vi "参数设置页.vi"() -> ()   [LabVIEW 2016, in "斯坦道氨氮.lvlib"]
uses:
  <vilib>/Plasmionique/MB Master/MB_Master/MB_Master.lvclass
  <vilib>/ptbypt/NI_PtbyPt.lvlib
panel:
  out "数据刷新时间":string
  in  "通讯连接":bool
  out "MB table":enum32{"Serial", "TCP"}(tab)
  in  "请选择串口:":refnum<visa-resource-name>
  in  "IP":string="127.0.0.1"
  in  "PORT":string="1001"
  in  "通信方式选择":enum16{"串口", "TCP"}(ring)
  in  "盐度自动补偿：":bool
  out "盐度补偿值":dbl caption="盐度补偿值："
  in  "刷新":bool
  in  "测量模式":enum16{"水样测量", "零点核查", "跨度核查", "标样核查", "加标回收"}(ring)
  in  "参数下拉列表":u16(ring)
  in  "量程下拉列表":enum16{"低量程", "高量程"}(ring)
  in  "流程路径":path=path "data/流程.xml"
  in  "标样核查量程模式":enum16{"高量程", "低量程", "自动"}(ring) caption="标样核查量程模式："
  in  "加标回收量程模式":enum16{"高量程", "低量程", "自动"}(ring) caption="加标回收量程模式："
  in  "跨度核查量程模式":enum16{"高量程", "低量程", "自动"}(ring) caption="跨度核查量程模式："
  in  "零点核查量程模式":enum16{"高量程", "低量程", "自动"}(ring) caption="零点核查量程模式："
  in  "水样测试量程模式":enum16{"高量程", "低量程", "自动"}(ring) caption="水样测试量程模式："
  out "稀释度":dbl caption="稀释度："
  out "阈值（高->低）":dbl caption="阈值（高->低）："
  out "阈值（低->高）":dbl caption="阈值（低->高）："
  out "量程下限":dbl caption="量程下限："
  out "量程上限":dbl caption="量程上限："
  out "检出限":dbl caption="检出限："
  out "曲线截距":dbl caption="曲线截距：" format="%#.6f"
  out "曲线斜率":dbl caption="曲线斜率：" format="%#.6f"
  out "二次多项式系数":dbl caption="二次多项式系数：" format="%#.6f"
  out "消解时长":dbl caption="消解时长："
  out "消解温度":dbl caption="消解温度："
  out "测量精度":u16 caption="测量精度："
  in  "标样核查标液浓度":dbl caption="标样核查标液浓度："
  in  "跨度核查标液浓度":dbl caption="跨度核查标液浓度："
  in  "零点核查标液浓度":dbl caption="零点核查标液浓度："
  in  "跨度值":dbl caption="跨度值："
  # "ppt"
  # "mg/L"
  # "mg/L"
  # "mg/L"
  # "mg/L"
  # "mg/L"
  # "min"
  # "℃"
  # "mg/L"
  # "mg/L"
  # "mg/L"
  # "mg/L"
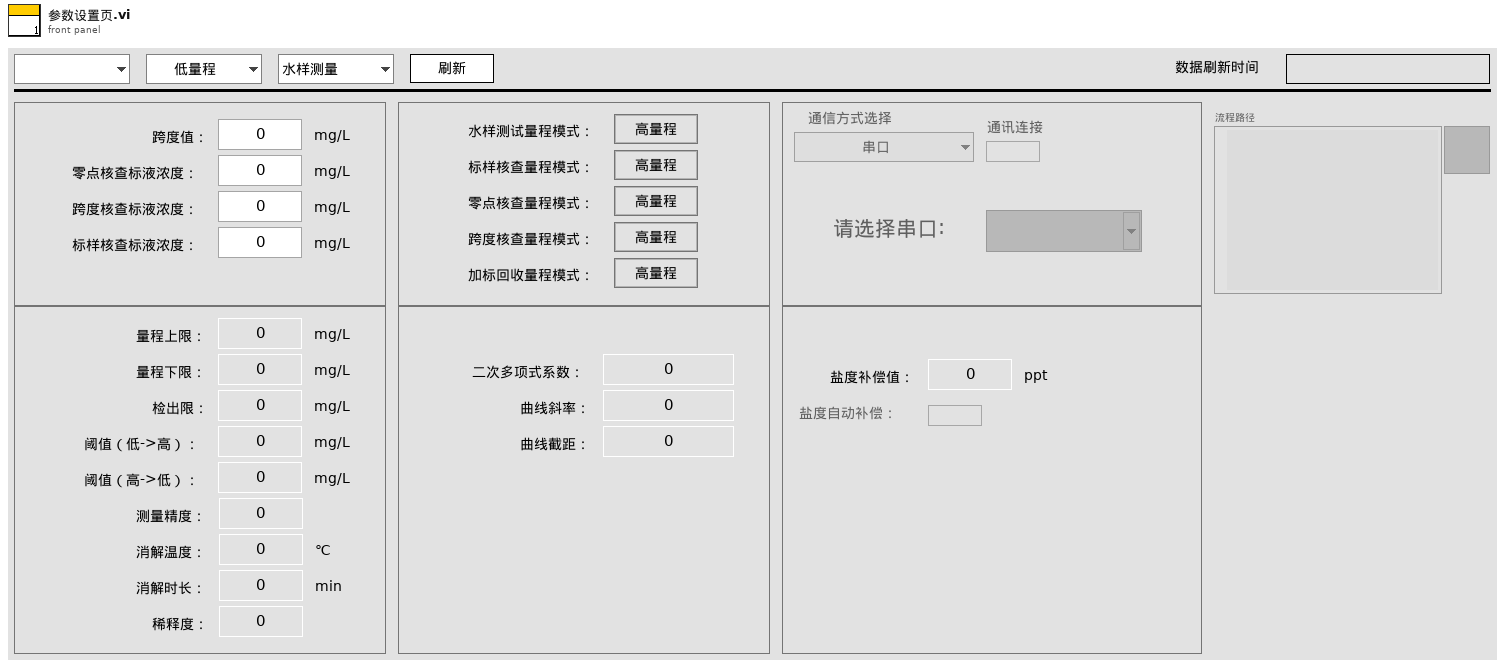
[diagram p1: front panel]
types:
  T1 = typedef "LVStringsAndValuesArrayTypeDef_U16.ctl" = cluster{"String":string, "Value":u16}[]
  T2 = enum8{"Enabled", "Disabled", "Disabled and Grayed Out"}
  T3 = cluster{"标液浓度1":dbl, "测量吸光度1":dbl, "样品1启用":bool, "标液浓度2":dbl, "测量吸光度2":dbl, "样品2启用":bool, "标液浓度3":dbl, "测量吸光度3":dbl, "样品3启用":bool, "标液浓度4":dbl, "测量吸光度4":dbl, "样品4启用":bool, "标液浓度5":dbl, "测量吸光度5":dbl, "样品5启用":bool, "模型":enum32{"线性", "多项式"}, "精度":dbl, "XY图":cluster{"X Values":dbl[], "Y Values":dbl[]}[], "拟合公式":string, "r^2":dbl, "标样一校准时间":timestamp, "标样二校准时间":timestamp, "标样三校准时间":timestamp, "标样四校准时间":timestamp, "标样五校准时间":timestamp, "二次方程":cluster{"c":dbl, "x":dbl, "x^2":dbl}, "标定时间":timestamp}
  T4 = cluster{"系统时间":timestamp, "工作状态":u16, "测量模式":enum16{"待机", "连续模式", "周期模式", "定点模式", "受控模式", "手动模式"}, "告警代码":u16, "故障代码":u16, "日志代码":u16, "软件版本":u16, "F0":sgl, "F1":sgl, "F2":sgl, "F3":sgl, "T":sgl, "H":sgl, "id":u16, "flowid":u16, "量程":u16, "总磷控温温度1":sgl, "营养盐控温温度2":sgl, "ADC":sgl}
  T5 = cluster{"测量精度":u16, "检出限":dbl, "上限":dbl, "下限":dbl, "阈值（低->高）":dbl, "阈值（高->低）":dbl, "稀释度":dbl}
  T6 = cluster{"泵类型":u8, "进样速度":u32, "出样速度":u32, "泵阀量":u8, "光谱仪类型":u8, "光谱采样次数":u8, "氙灯次数":u8, "B":u16, "C":u16, "D":u16, "E":u16, "B_COD":u16, "C_COD":u16, "D_COD":u16, "E_COD":u16, "G":u16, "M":u16, "N":u16, "氨氮注射泵控温下限":sgl, "氨氮注射泵控温上限":sgl, "总氮注射泵控温下限":sgl, "总氮注射泵控温上限":sgl, "消解温度下限":sgl, "消解温度上限":sgl, "加热10s限值":sgl, "高温高压阀开阀温度":sgl, "总氮x公式0":u8, "总氮x公式1":sgl, "总氮x公式2":sgl, "总磷浊度稀释系数":sgl, "总磷浊度补偿权重1":sgl, "总磷浊度补偿权重2":sgl, "盐度系数":sgl, "氨氮补偿系数1":sgl, "氨氮补偿系数2":sgl}
  T7 = cluster{"标液浓度1":dbl, "测量吸光度1":dbl, "样品1启用":bool, "标液浓度2":dbl, "测量吸光度2":dbl, "样品2启用":bool, "标液浓度3":dbl, "测量吸光度3":dbl, "样品3启用":bool, "标液浓度4":dbl, "测量吸光度4":dbl, "样品4启用":bool, "标液浓度5":dbl, "测量吸光度5":dbl, "样品5启用":bool, "模型":enum32{"线性", "多项式"}, "精度":dbl, "XY图":cluster{"X Values":dbl[], "Y Values":dbl[]}[], "拟合公式":string, "r^2":dbl, "标样一校准时间":timestamp, "标样二校准时间":timestamp, "标样三校准时间":timestamp, "标样四校准时间":timestamp, "标样五校准时间":timestamp, "二次方程":cluster{"c":dbl, "x":dbl, "x^2":dbl}, "标定时间":timestamp}[][]
  T8 = typedef "斯坦道氨氮.lvlib/关键参数.ctl" = cluster{"测量量程":sgl, "测量检出限":sgl, "测量精度":sgl, "测量间隔":sgl, "消解温度":sgl, "消解时长":sgl, "三项式系数":sgl, "二次多项式系数":sgl, "曲线斜率":sgl, "曲线截距":sgl, "线性相关系数":sgl, "空白校准时间":timestamp, "标样校准时间":timestamp, "测量信号值":sgl, "稀释倍数":sgl, "量程系数":sgl}
  T9 = cluster{"水样测试量程模式":enum16{"高量程", "低量程", "自动"}, "零点核查量程模式":enum16{"高量程", "低量程", "自动"}, "跨度核查量程模式":enum16{"高量程", "低量程", "自动"}, "加标回收量程模式":enum16{"高量程", "低量程", "自动"}, "标样核查量程模式":enum16{"高量程", "低量程", "自动"}}
  T10 = cluster{"总磷跨度值":dbl, "总磷零点标准液浓度":dbl, "总磷跨度标准液浓度":dbl, "总磷标准液标准浓度":dbl, "总氮跨度值":dbl, "总氮零点标准液浓度":dbl, "总氮跨度标准液浓度":dbl, "总氮标准液标准浓度":dbl, "COD跨度值":dbl, "COD零点标准液浓度":dbl, "COD跨度标准液浓度":dbl, "COD标准液标准浓度":dbl, "氨氮跨度值":dbl, "氨氮零点标准液浓度":dbl, "氨氮跨度标准液浓度":dbl, "氨氮标准液标准浓度":dbl, "磷酸盐跨度值":dbl, "磷酸盐零点标准液浓度":dbl, "磷酸盐跨度标准液浓度":dbl, "磷酸盐标准液标准浓度":dbl, "硝氮跨度值":dbl, "硝氮零点标准液浓度":dbl, "硝氮跨度标准液浓度":dbl, "硝氮标准液标准浓度":dbl, "亚硝氮跨度值":dbl, "亚硝氮零点标准液浓度":dbl, "亚硝氮跨度标准液浓度":dbl, "亚硝氮标准液标准浓度":dbl, "硫化物跨度值":dbl, "硫化物零点标准液浓度":dbl, "硫化物跨度标准液浓度":dbl, "硫化物标准液标准浓度":dbl, "硅酸盐跨度值":dbl, "硅酸盐零点标准液浓度":dbl, "硅酸盐跨度标准液浓度":dbl, "硅酸盐标准液标准浓度":dbl}
  T11 = cluster{"水样测试量程模式":u16, "零点核查量程模式":u16, "跨度核查量程模式":u16, "加标回收量程模式":u16, "标样核查量程模式":u16}
  T12 = cluster{"水样测试量程模式":enum16{"H", "L", "AUTO"}, "空白核查量程模式":enum16{"H", "L", "AUTO"}, "跨度核查量程模式":enum16{"H", "L", "AUTO"}, "加标回收量程模式":enum16{"H", "L", "AUTO"}, "标样核查量程模式":enum16{"H", "L", "AUTO"}}
  T13 = cluster{"水样测试量程模式":u16, "空白核查量程模式":u16, "跨度核查量程模式":u16, "加标回收量程模式":u16, "标样核查量程模式":u16}
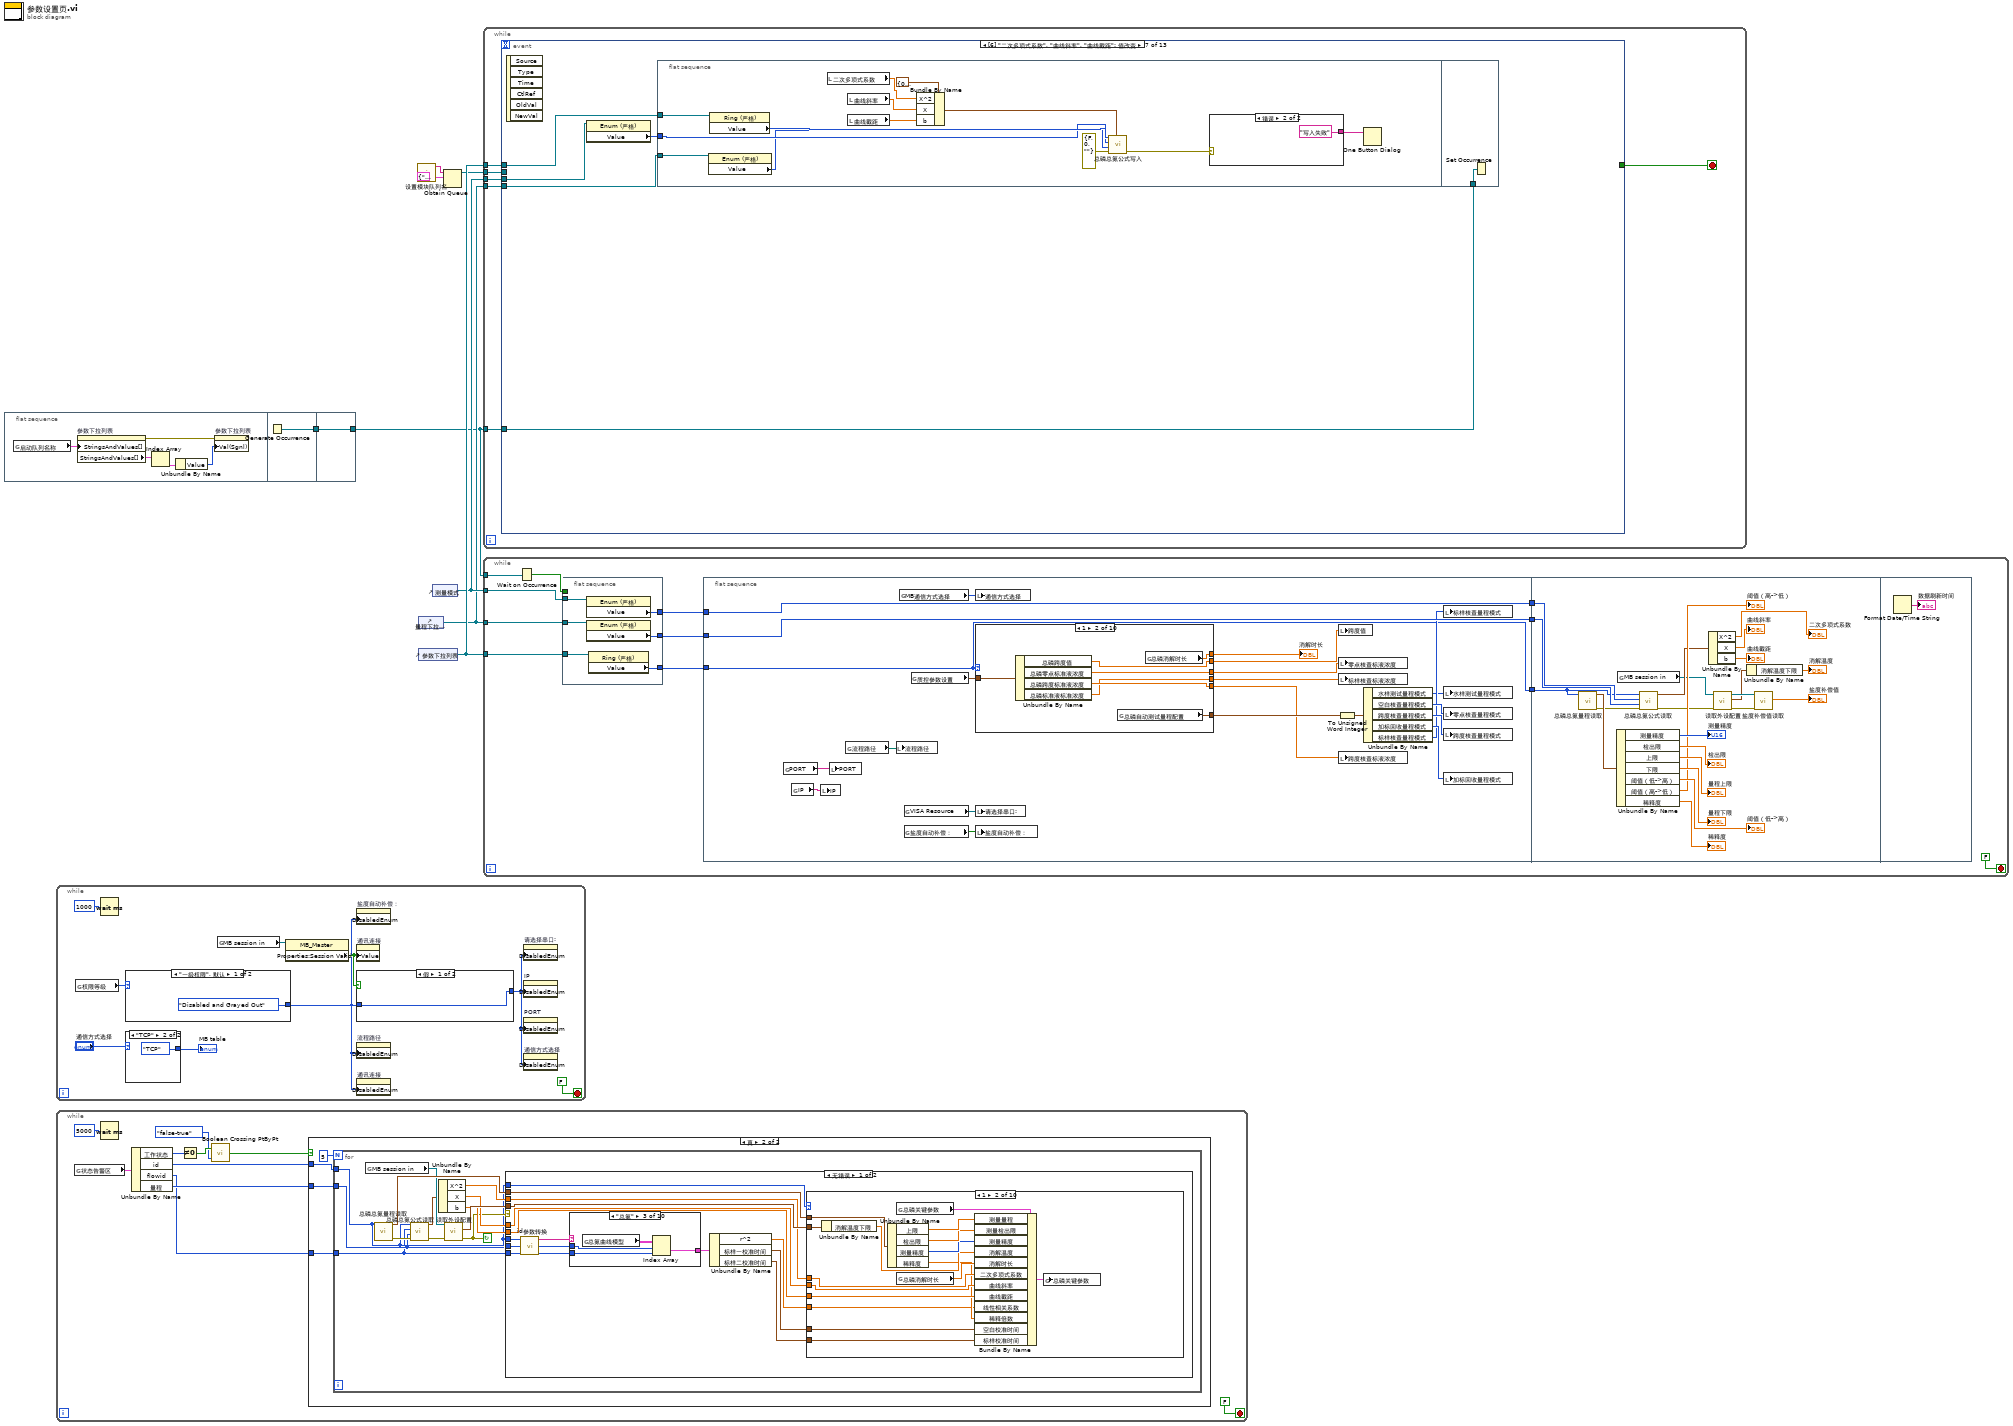
[diagram p0: block diagram]
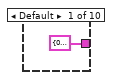
[diagram p3: hidden frame]
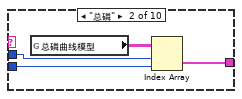
[diagram p4: hidden frame]
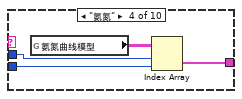
[diagram p5: hidden frame]
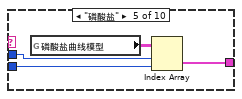
[diagram p6: hidden frame]
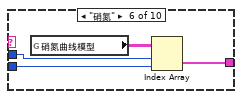
[diagram p7: hidden frame]
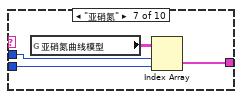
[diagram p8: hidden frame]
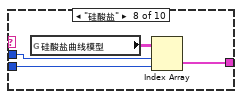
[diagram p9: hidden frame]
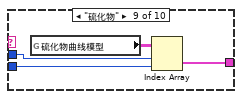
[diagram p10: hidden frame]
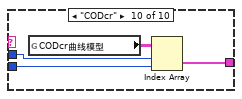
[diagram p11: hidden frame]
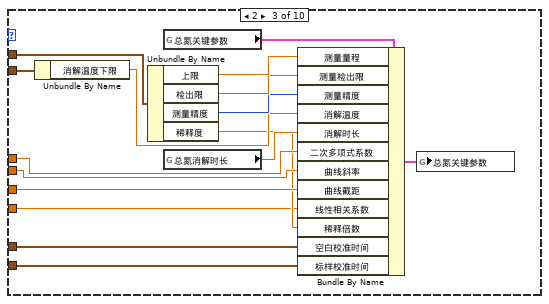
[diagram p13: hidden frame]
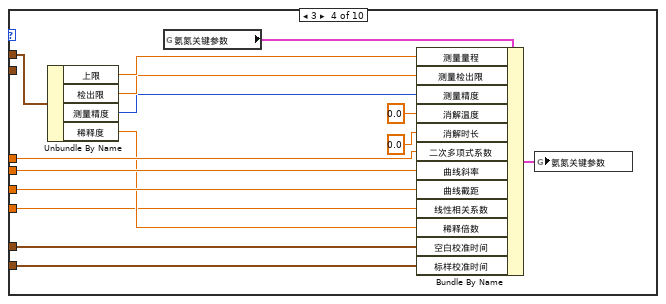
[diagram p14: hidden frame]
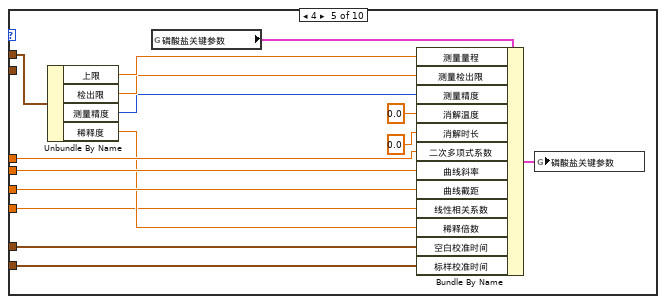
[diagram p15: hidden frame]
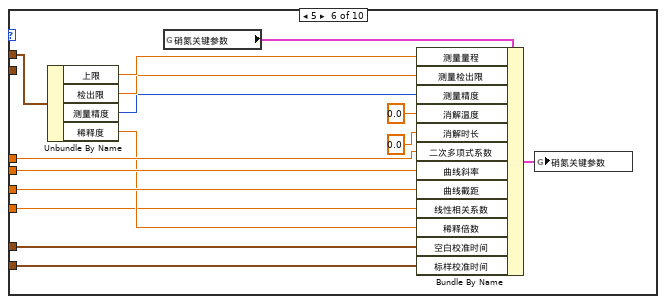
[diagram p16: hidden frame]
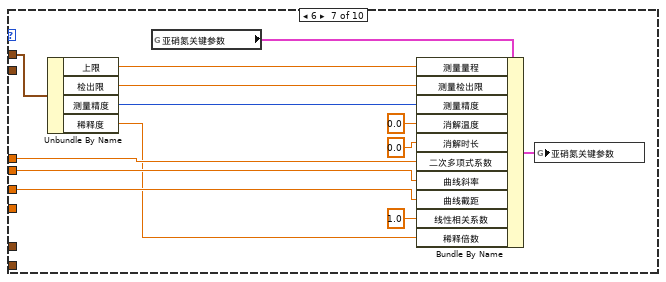
[diagram p17: hidden frame]
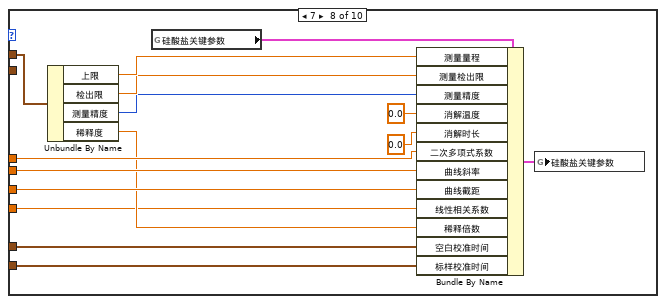
[diagram p18: hidden frame]
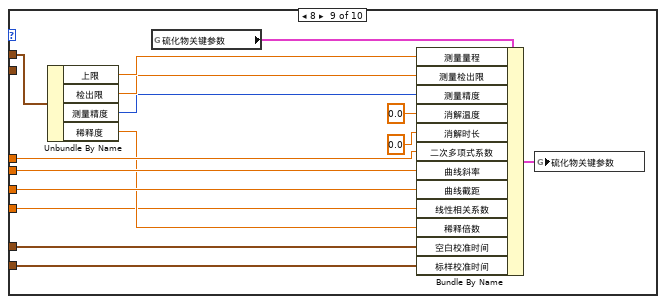
[diagram p19: hidden frame]
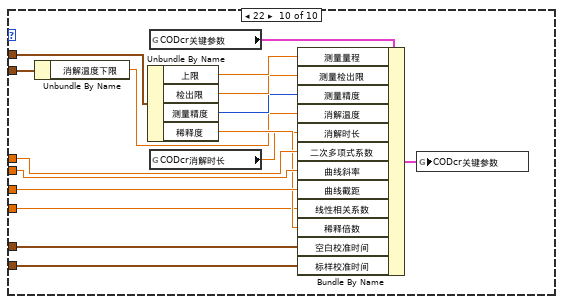
[diagram p20: hidden frame]
diagram:
  n1 = flat-sequence {
    tunnel: [w14] -> w7
    tunnel: [w15] -> w1
    tunnel: w7 -> [w15]
    frame #0 {
      n2 = global read "总磷总氮断电保存全局变量.vi" "启动队列名称"() -> (w9:cluster{"String":string, "Value":u16}[])
      n3 = property on="参数下拉列表" class="Ring (严格)"("StringsAndValues[]"=w9) -> (error out=w12:errorcluster, "StringsAndValues[]"=w10:T1)  [unwired: 2 in, 1 out]
      n4 = Index Array(array=w10) -> (element=w11:cluster{"String":string, "Value":u16})  [unwired: 1 in]
      n5 = Unbundle By Name(w11) -> ("Value"=w13:u16)
      n6 = property on="参数下拉列表" class="Ring (严格)"(error in=w12, "Val(Sgnl)"=w13) -> ()  [unwired: 1 in, 2 out]
    }
    frame #1 {
      n7 = Generate Occurrence() -> (w14:refnum<k4>)
    }
    frame #2 {
    }
  }
  n8 = while {
    stop <- FALSE stop-if-true
    n9 = global read "VAR总磷总氮全局变量.vi" "权限等级"() -> (w16:enum16{"一级权限", "二级权限", "三级权限", "超级权限"})
    n10 = Wait (ms)(milliseconds to wait=u32 1000 ("等待时间（毫秒）")) -> ()  [unwired: 1 out]
    n11 = case shown="\"一级权限\", 默认" w16 {
      tunnel: [T2."Disabled and Grayed Out" ("禁用") T2."Enabled" ("禁用")] -> w17
      frame "一级权限", Default {
      }
      frame "二级权限".."超级权限" {
      }
    }
    n12 = case shown="\"TCP\"" "通信方式选择" {
      tunnel: [enum32{"Serial", "TCP"}."Serial" ("MB table") enum32{"Serial", "TCP"}."TCP" ("MB table")] -> w19
      frame "串口", Default {
      }
      frame "TCP" {
      }
    }
    "MB table" <- w19
    n13 = global read "VAR总磷总氮全局变量.vi" "MB session in"() -> (w23:refnum<class "MB_Master.lvclass">)
    n14 = property class="MB_Master"(reference=w23) -> ("Properties:Session Valid"=w21:bool)  [unwired: 1 in, 2 out]
    n15 = property on="盐度自动补偿：" class="Bool (严格)"("DisabledEnum"=w17) -> ()  [unwired: 2 in, 2 out]
    n16 = property on="通讯连接" class="Bool (严格)"("Value"=w21) -> ()  [unwired: 2 in, 2 out]
    n17 = case shown="假" w21 {
      tunnel: [w29 T2."Disabled and Grayed Out" ("禁用")] -> w20
      tunnel: w17 -> [w29 _]
      frame False {
      }
      frame True {
      }
    }
    n18 = property on="流程路径" class="Path"("DisabledEnum"=w17) -> ()  [unwired: 2 in, 2 out]
    n19 = property on="通讯连接" class="Bool (严格)"("DisabledEnum"=w17) -> ()  [unwired: 2 in, 2 out]
    n20 = property on="请选择串口:" class="VISAName"("DisabledEnum"=w20) -> ()  [unwired: 2 in, 2 out]
    n21 = property on="IP" class="Str"("DisabledEnum"=w20) -> ()  [unwired: 2 in, 2 out]
    n22 = property on="PORT" class="Str"("DisabledEnum"=w20) -> ()  [unwired: 2 in, 2 out]
    n23 = property on="通信方式选择" class="Enum (严格)"("DisabledEnum"=w20) -> ()  [unwired: 2 in, 2 out]
  }
  n24 = while {
    stop <- FALSE stop-if-true
    n25 = global read "VAR总磷总氮全局变量.vi" "状态告警区"() -> (w40:T4)
    n26 = Wait (ms)(milliseconds to wait=u32 5000 ("等待时间（毫秒）")) -> ()  [unwired: 1 out]
    n27 = Unbundle By Name(w40) -> ("工作状态"=w36:u16, "id"=w37:u16, "flowid"=w38:u16, "量程"=w39:u16)
    n28 = Not Equal To 0?(x=w36) -> (x != 0?=w35:bool)
    n29 = call <vilib>:"Boolean Crossing PtByPt.vi"("direction"=enum16{"either", "false-true", "true-false"}."false-true", "input"=w35) -> ("crossing"=w33:bool)  [unwired: 1 in]
    n30 = case shown="真" w33 {
      tunnel: w39 -> [_ w44]
      tunnel: w38 -> [_ w43]
      tunnel: w37 -> [_ w42]
      frame False {
      }
      frame True {
        n31 = for {
          N: 5 -> [_]
          tunnel: w44 -> [w46]
          tunnel: w43 -> [w45]
          tunnel: w42 -> [w47]
          stop <- w48 continue-if-true
          n32 = global read "VAR总磷总氮全局变量.vi" "MB session in"() -> (w56:refnum<class "MB_Master.lvclass">)
          n33 = call "总磷总氮量程读取.vi"("测量参数"=w47) -> ("error out"=w50:errorcluster, "量程参数读取"=w57:T5)  [unwired: 9 in]
          n34 = call "总磷总氮公式读取.vi"("error in (no error)"=w50, "量程"=w46, "测量模式"=w45, "测量参数"=w47) -> ("error out"=w49:errorcluster, "公式"=w54:cluster{"X^2":dbl, "X":dbl, "b":dbl})  [unwired: 6 in]
          n35 = Unbundle By Name(w54) -> ("X^2"=w53:dbl, "X"=w52:dbl, "b"=w51:dbl)
          n36 = call "读取外设配置.vi"("error in (no error)"=w49, "MB session in"=w56) -> ("error out"=w48:errorcluster, "外设配置"=w55:T6)  [unwired: 7 in, 1 out]
          n37 = case shown="无错误" w48 {
            tunnel: w57 -> [w71 _]
            tunnel: w55 -> [w70 _]
            tunnel: w53 -> [w69 _]
            tunnel: w52 -> [w68 _]
            tunnel: w51 -> [w67 _]
            tunnel: w47 -> [w66 _]
            tunnel: w47 -> [w63 _]
            tunnel: w46 -> [w62 _]
            tunnel: w45 -> [w61 _]
            frame No Error {
              n38 = call "id参数转换.vi"("id"=w63) -> ("table输出"=w65:string)  [unwired: 9 in, 1 out]
              n39 = case shown="\"总氮\"" w65 {
                tunnel: w61 -> [_ w75 w77 w82 w86 w90 w94 w98 w102 w106]
                tunnel: w62 -> [_ w76 w78 w83 w87 w91 w95 w99 w103 w107]
                tunnel: [T3 {"标液浓度1"=0.0, "测量吸光度1"=0.0, "样品1启用"=FALSE, "标液浓度2"=0.0, "测量吸光度2"=0.0, "样品2启用"=FALSE, "标液浓度3"=0.0, "测量吸光度3"=0.0, "样品3启用"=FALSE, "标液浓度4"=0.0, "测量吸光度4"=0.0, "样品4启用"=FALSE, "标液浓度5"=0.0, "测量吸光度5"=0.0, "样品5启用"=FALSE, "模型"=enum."线性", "精度"=0.0, "XY图"=[], "拟合公式"="", "r^2"=0.0, "标样一校准时间"=timestamp(0 s since 1904-01-01), "标样二校准时间"=timestamp(0 s since 1904-01-01), "标样三校准时间"=timestamp(0 s since 1904-01-01), "标样四校准时间"=timestamp(0 s since 1904-01-01), "标样五校准时间"=timestamp(0 s since 1904-01-01), "二次方程"={"c"=0.0, "x"=0.0, "x^2"=0.0}, "标定时间"=timestamp(0 s since 1904-01-01)} ("总磷曲线模型") w73 w79 w81 w85 w89 w93 w97 w101 w105] -> w64
                frame Default {
                }
                frame "总磷" {
                  n40 = global read "校准数据全局变量.vi" "总磷曲线模型"() -> (w74:T7)
                  n41 = Index Array(array=w74, index (row)=w76, index (col)=w75) -> (element=w73:T3)
                }
                frame "总氮" {
                  n42 = global read "校准数据全局变量.vi" "总氮曲线模型"() -> (w80:T7)
                  n43 = Index Array(array=w80, index (row)=w78, index (col)=w77) -> (element=w79:T3)
                }
                frame "氨氮" {
                  n44 = global read "校准数据全局变量.vi" "氨氮曲线模型"() -> (w84:T7)
                  n45 = Index Array(array=w84, index (row)=w83, index (col)=w82) -> (element=w81:T3)
                }
                frame "磷酸盐" {
                  n46 = global read "校准数据全局变量.vi" "磷酸盐曲线模型"() -> (w88:T7)
                  n47 = Index Array(array=w88, index (row)=w87, index (col)=w86) -> (element=w85:T3)
                }
                frame "硝氮" {
                  n48 = global read "校准数据全局变量.vi" "硝氮曲线模型"() -> (w92:T7)
                  n49 = Index Array(array=w92, index (row)=w91, index (col)=w90) -> (element=w89:T3)
                }
                frame "亚硝氮" {
                  n50 = global read "校准数据全局变量.vi" "亚硝氮曲线模型"() -> (w96:T7)
                  n51 = Index Array(array=w96, index (row)=w95, index (col)=w94) -> (element=w93:T3)
                }
                frame "硅酸盐" {
                  n52 = global read "校准数据全局变量.vi" "硅酸盐曲线模型"() -> (w100:T7)
                  n53 = Index Array(array=w100, index (row)=w99, index (col)=w98) -> (element=w97:T3)
                }
                frame "硫化物" {
                  n54 = global read "校准数据全局变量.vi" "硫化物曲线模型"() -> (w104:T7)
                  n55 = Index Array(array=w104, index (row)=w103, index (col)=w102) -> (element=w101:T3)
                }
                frame "CODcr" {
                  n56 = global read "校准数据全局变量.vi" "CODcr曲线模型"() -> (w108:T7)
                  n57 = Index Array(array=w108, index (row)=w107, index (col)=w106) -> (element=w105:T3)
                }
              }
              n58 = Unbundle By Name(w64) -> ("r^2"=w60:dbl, "标样一校准时间"=w59:timestamp, "标样二校准时间"=w58:timestamp)
              n59 = case shown="1" w66 {
                tunnel: w71 -> [_ w122 w138 w153 w168 w183 w196 w211 w226 w242]
                tunnel: w70 -> [_ w118 w134 _ _ _ _ _ _ w234]
                tunnel: w69 -> [_ w115 w131 w149 w164 w179 w192 w207 w222 w238]
                tunnel: w68 -> [_ w114 w130 w148 w163 w178 w191 w206 w221 w237]
                tunnel: w67 -> [_ w113 w129 w147 w162 w177 w190 w205 w220 w236]
                tunnel: w60 -> [_ w109 w127 w143 w156 w173 _ w201 w214 w231]
                tunnel: w59 -> [_ w110 w126 w142 w158 w172 _ w200 w216 w230]
                tunnel: w58 -> [_ w111 w125 w141 w157 w171 _ w199 w215 w229]
                frame 0, Default {
                }
                frame 1 {
                  n60 = Unbundle By Name(w118) -> ("消解温度下限"=w117:sgl)
                  n61 = Unbundle By Name(w122) -> ("上限"=w121:dbl, "检出限"=w120:dbl, "测量精度"=w119:u16, "稀释度"=w112:dbl)
                  n62 = global read "VAR总磷总氮全局变量.vi" "总磷关键参数"() -> (w123:T8)
                  n63 = global read "总磷总氮断电保存全局变量.vi" "总磷消解时长"() -> (w116:dbl)
                  n64 = Bundle By Name(cluster=w123, "测量量程"=w121, "测量检出限"=w120, "测量精度"=w119, "消解温度"=w117, "消解时长"=w116, "二次多项式系数"=w115, "曲线斜率"=w114, "曲线截距"=w113, "线性相关系数"=w109, "稀释倍数"=w112, "空白校准时间"=w110, "标样校准时间"=w111) -> (w124:T8)
                  n65 = global write "VAR总磷总氮全局变量.vi" "总磷关键参数"(w124) -> ()
                }
                frame 2 {
                  n66 = Unbundle By Name(w134) -> ("消解温度下限"=w133:sgl)
                  n67 = Unbundle By Name(w138) -> ("上限"=w137:dbl, "检出限"=w136:dbl, "测量精度"=w135:u16, "稀释度"=w128:dbl)
                  n68 = global read "VAR总磷总氮全局变量.vi" "总氮关键参数"() -> (w139:T8)
                  n69 = global read "总磷总氮断电保存全局变量.vi" "总氮消解时长"() -> (w132:dbl)
                  n70 = Bundle By Name(cluster=w139, "测量量程"=w137, "测量检出限"=w136, "测量精度"=w135, "消解温度"=w133, "消解时长"=w132, "二次多项式系数"=w131, "曲线斜率"=w130, "曲线截距"=w129, "线性相关系数"=w127, "稀释倍数"=w128, "空白校准时间"=w126, "标样校准时间"=w125) -> (w140:T8)
                  n71 = global write "VAR总磷总氮全局变量.vi" "总氮关键参数"(w140) -> ()
                }
                frame 3 {
                  n72 = Unbundle By Name(w153) -> ("上限"=w152:dbl, "检出限"=w151:dbl, "测量精度"=w150:u16, "稀释度"=w146:dbl)
                  n73 = global read "VAR总磷总氮全局变量.vi" "氨氮关键参数"() -> (w154:T8)
                  n74 = Bundle By Name(cluster=w154, "测量量程"=w152, "测量检出限"=w151, "测量精度"=w150, "消解温度"=sgl 0.0, "消解时长"=sgl 0.0, "二次多项式系数"=w149, "曲线斜率"=w148, "曲线截距"=w147, "线性相关系数"=w143, "稀释倍数"=w146, "空白校准时间"=w142, "标样校准时间"=w141) -> (w155:T8)
                  n75 = global write "VAR总磷总氮全局变量.vi" "氨氮关键参数"(w155) -> ()
                }
                frame 4 {
                  n76 = Unbundle By Name(w168) -> ("上限"=w167:dbl, "检出限"=w166:dbl, "测量精度"=w165:u16, "稀释度"=w161:dbl)
                  n77 = global read "VAR总磷总氮全局变量.vi" "磷酸盐关键参数"() -> (w169:T8)
                  n78 = Bundle By Name(cluster=w169, "测量量程"=w167, "测量检出限"=w166, "测量精度"=w165, "消解温度"=sgl 0.0, "消解时长"=sgl 0.0, "二次多项式系数"=w164, "曲线斜率"=w163, "曲线截距"=w162, "线性相关系数"=w156, "稀释倍数"=w161, "空白校准时间"=w158, "标样校准时间"=w157) -> (w170:T8)
                  n79 = global write "VAR总磷总氮全局变量.vi" "磷酸盐关键参数"(w170) -> ()
                }
                frame 5 {
                  n80 = Unbundle By Name(w183) -> ("上限"=w182:dbl, "检出限"=w181:dbl, "测量精度"=w180:u16, "稀释度"=w176:dbl)
                  n81 = global read "VAR总磷总氮全局变量.vi" "硝氮关键参数"() -> (w184:T8)
                  n82 = Bundle By Name(cluster=w184, "测量量程"=w182, "测量检出限"=w181, "测量精度"=w180, "消解温度"=sgl 0.0, "消解时长"=sgl 0.0, "二次多项式系数"=w179, "曲线斜率"=w178, "曲线截距"=w177, "线性相关系数"=w173, "稀释倍数"=w176, "空白校准时间"=w172, "标样校准时间"=w171) -> (w185:T8)
                  n83 = global write "VAR总磷总氮全局变量.vi" "硝氮关键参数"(w185) -> ()
                }
                frame 6 {
                  n84 = Unbundle By Name(w196) -> ("上限"=w195:dbl, "检出限"=w194:dbl, "测量精度"=w193:u16, "稀释度"=w188:dbl)
                  n85 = global read "VAR总磷总氮全局变量.vi" "亚硝氮关键参数"() -> (w197:T8)
                  n86 = Bundle By Name(cluster=w197, "测量量程"=w195, "测量检出限"=w194, "测量精度"=w193, "消解温度"=sgl 0.0, "消解时长"=sgl 0.0, "二次多项式系数"=w192, "曲线斜率"=w191, "曲线截距"=w190, "线性相关系数"=sgl 1.0, "稀释倍数"=w188) -> (w198:T8)
                  n87 = global write "VAR总磷总氮全局变量.vi" "亚硝氮关键参数"(w198) -> ()
                }
                frame 7 {
                  n88 = Unbundle By Name(w211) -> ("上限"=w210:dbl, "检出限"=w209:dbl, "测量精度"=w208:u16, "稀释度"=w204:dbl)
                  n89 = global read "VAR总磷总氮全局变量.vi" "硅酸盐关键参数"() -> (w212:T8)
                  n90 = Bundle By Name(cluster=w212, "测量量程"=w210, "测量检出限"=w209, "测量精度"=w208, "消解温度"=sgl 0.0, "消解时长"=sgl 0.0, "二次多项式系数"=w207, "曲线斜率"=w206, "曲线截距"=w205, "线性相关系数"=w201, "稀释倍数"=w204, "空白校准时间"=w200, "标样校准时间"=w199) -> (w213:T8)
                  n91 = global write "VAR总磷总氮全局变量.vi" "硅酸盐关键参数"(w213) -> ()
                }
                frame 8 {
                  n92 = Unbundle By Name(w226) -> ("上限"=w225:dbl, "检出限"=w224:dbl, "测量精度"=w223:u16, "稀释度"=w219:dbl)
                  n93 = global read "VAR总磷总氮全局变量.vi" "硫化物关键参数"() -> (w227:T8)
                  n94 = Bundle By Name(cluster=w227, "测量量程"=w225, "测量检出限"=w224, "测量精度"=w223, "消解温度"=sgl 0.0, "消解时长"=sgl 0.0, "二次多项式系数"=w222, "曲线斜率"=w221, "曲线截距"=w220, "线性相关系数"=w214, "稀释倍数"=w219, "空白校准时间"=w216, "标样校准时间"=w215) -> (w228:T8)
                  n95 = global write "VAR总磷总氮全局变量.vi" "硫化物关键参数"(w228) -> ()
                }
                frame 22 {
                  n96 = Unbundle By Name(w234) -> ("消解温度下限"=w233:sgl)
                  n97 = Unbundle By Name(w242) -> ("上限"=w241:dbl, "检出限"=w240:dbl, "测量精度"=w239:u16, "稀释度"=w235:dbl)
                  n98 = global read "VAR总磷总氮全局变量.vi" "CODcr关键参数"() -> (w243:T8)
                  n99 = global read "总磷总氮断电保存全局变量.vi" "CODcr消解时长"() -> (w232:dbl)
                  n100 = Bundle By Name(cluster=w243, "测量量程"=w241, "测量检出限"=w240, "测量精度"=w239, "消解温度"=w233, "消解时长"=w232, "二次多项式系数"=w238, "曲线斜率"=w237, "曲线截距"=w236, "线性相关系数"=w231, "稀释倍数"=w235, "空白校准时间"=w230, "标样校准时间"=w229) -> (w244:T8)
                  n101 = global write "VAR总磷总氮全局变量.vi" "CODcr关键参数"(w244) -> ()
                }
              }
            }
            frame Error {
            }
          }
        }
      }
    }
  }
  n102 = call "设置模块队列名.vi"() -> ("Msg"=w5:string)  [unwired: 5 in]
  n103 = control-ref of="量程下拉列表"() -> (w2:refnum<vi>)
  n104 = control-ref of="参数下拉列表"() -> (w8:refnum<vi>)
  n105 = control-ref of="测量模式"() -> (w3:refnum<vi>)
  n106 = Obtain Queue(name (unnamed)=w5, element data type=cluster{"命令":string, "data":variant} {"命令"="", "data"=variant}) -> (queue out=w4:refnum<queue>)  [unwired: 3 in, 2 out]
  n107 = while {
    tunnel: w1 -> [w249]
    tunnel: w8 -> [w248]
    tunnel: w4 -> [w247]
    tunnel: w3 -> [w246]
    tunnel: w2 -> [w245]
    stop <- w250 stop-if-true
    n108 = event shown="[6] \"二次多项式系数\", \"曲线斜率\", \"曲线截距\": 值改变" {
      selector: _ -> [_ _ _ _ _ _ _ _ _ _ _ _ _]
      dyn-events: _ -> [_ _ _ _ _ _ _ _ _ _ _ _ _]
      timeout: _ -> [_ _ _ _ _ _ _ _ _ _ _ _ _]
      tunnel: [_ TRUE _ _ _ _ _ _ _ _ _ _ _] -> w250
      tunnel: w249 -> [_ _ w252 _ _ _ w283 _ _ _ _ w326 _]
      tunnel: w248 -> [_ _ _ _ w271 _ w287 _ _ _ _ w328 _]
      tunnel: w247 -> [_ _ _ _ _ _ _ _ _ _ _ _ w418]
      tunnel: w246 -> [_ _ _ _ _ _ w286 _ _ _ _ _ _]
      tunnel: w245 -> [_ _ _ _ _ _ w284 _ _ _ _ _ _]
      event Timeout {
        n109 = event-data() -> ()  [unwired: 1 in, 3 out]
      }
      event Panel Close {
        n110 = event-data() -> ()  [unwired: 1 in, 4 out]
      }
      event "参数下拉列表", "量程下拉列表", "测量模式", "刷新": Value Change {
        n111 = event-data() -> ()  [unwired: 1 in, 6 out]
        n112 = Set Occurrence(w252) -> ()
      }
      event "跨度值", "零点核查标液浓度", "跨度核查标液浓度", "标样核查标液浓度", "消解温度", "消解时长", "检出限", "量程上限", "量程下限", "阈值（低->高）", "阈值（高->低）", "稀释度": Mouse Down {
        n113 = event-data() -> ("CtlRef"=w254:refnum<vi>)  [unwired: 1 in, 5 out]
        n114 = global read "VAR总磷总氮全局变量.vi" "权限等级"() -> (w253:enum16{"一级权限", "二级权限", "三级权限", "超级权限"})
        n115 = case shown="\"二级权限\"..\"超级权限\"" w253 {
          tunnel: w254 -> [_ w258]
          frame "一级权限", Default {
          }
          frame "二级权限".."超级权限" {
            n116 = property class="DigNum (严格)"(reference=w258) -> (reference out=w256:refnum<vi>, "Value"=w257:dbl)  [unwired: 1 in, 1 out]
            n117 = call "数字键盘.vi"("OldNumber"=w257) -> ("NewNumber"=w255:dbl)
            n118 = property class="DigNum (严格)"(reference=w256, "Val(Sgnl)"=w255) -> ()  [unwired: 1 in, 2 out]
          }
        }
      }
      event "测量精度", "检出限", "量程上限", "量程下限", "阈值（低->高）", "阈值（高->低）", "稀释度": Value Change {
        n119 = event-data() -> ()  [unwired: 1 in, 6 out]
        n120 = property class="Ring (严格)"(reference=w271) -> ("Value"=w270:u16)  [unwired: 1 in, 2 out]
        n121 = local read "阈值（低->高）"() -> (w264:dbl)
        n122 = local read "阈值（高->低）"() -> (w263:dbl)
        n123 = local read "测量精度"() -> (w261:u16)
        n124 = local read "量程上限"() -> (w267:dbl)
        n125 = local read "量程下限"() -> (w266:dbl)
        n126 = local read "检出限"() -> (w265:dbl)
        n127 = local read "稀释度"() -> (w262:dbl)
        n128 = Bundle By Name(cluster=T5 {"测量精度"=0, "检出限"=0.0, "上限"=0.0, "下限"=0.0, "阈值（低->高）"=0.0, "阈值（高->低）"=0.0, "稀释度"=0.0} ("量程参数写入"), "测量精度"=w261, "检出限"=w265, "上限"=w267, "下限"=w266, "阈值（低->高）"=w264, "阈值（高->低）"=w263, "稀释度"=w262) -> (w268:T5)
        n129 = call "总磷总氮量程写入.vi"("量程参数写入"=w268, "测量参数"=w270) -> ("error out"=w259:errorcluster)  [unwired: 8 in]
        n130 = case shown="错误" w259 {
          tunnel: ["写入成功" "写入失败"] -> w260
          frame No Error {
          }
          frame Error {
          }
        }
        n131 = One Button Dialog(message=w260) -> ()  [unwired: 1 in, 1 out]
      }
      event "消解温度": Value Change {
        n132 = event-data() -> ("NewVal"=w276:dbl)  [unwired: 1 in, 5 out]
        n133 = global read "VAR总磷总氮全局变量.vi" "MB session in"() -> (w277:refnum<class "MB_Master.lvclass">)
        n134 = call "读取外设配置.vi"("MB session in"=w277) -> ("error out"=w280:errorcluster, "外设配置"=w279:T6)  [unwired: 8 in, 1 out]
        n135 = Bundle By Name(cluster=w279, "消解温度下限"=w276) -> (w278:T6)
        n136 = call "写入外设配置.vi"("error in (no error)"=w280, "外设配置"=w278, "MB session in"=w277) -> ("error out"=w275:errorcluster)  [unwired: 7 in, 1 out]
        n137 = case shown="错误" w275 {
          tunnel: ["写入成功" "写入失败"] -> w274
          frame No Error {
          }
          frame Error {
          }
        }
        n138 = One Button Dialog(message=w274) -> ()  [unwired: 1 in, 1 out]
      }
      event "二次多项式系数", "曲线斜率", "曲线截距": Value Change {
        n139 = event-data() -> ()  [unwired: 1 in, 6 out]
        n140 = property class="Enum (严格)"(reference=w286) -> ("Value"=w285:enum16{"水样测量", "零点核查", "跨度核查", "标样核查", "加标回收"})  [unwired: 1 in, 2 out]
        n141 = flat-sequence {
          tunnel: w287 -> [w300]
          tunnel: w285 -> [w298]
          tunnel: w284 -> [w297]
          tunnel: w283 -> [w303]
          frame #0 {
            n142 = property class="Enum (严格)"(reference=w297) -> ("Value"=w296:enum16{"低量程", "高量程"})  [unwired: 1 in, 2 out]
            n143 = property class="Ring (严格)"(reference=w300) -> ("Value"=w299:u16)  [unwired: 1 in, 2 out]
            n144 = local read "二次多项式系数"() -> (w293:dbl)
            n145 = local read "曲线斜率"() -> (w292:dbl)
            n146 = local read "曲线截距"() -> (w291:dbl)
            n147 = Bundle By Name(cluster=cluster{"X^2":dbl, "X":dbl, "b":dbl} {"X^2"=0.0, "X"=0.0, "b"=0.0} ("公式"), "X^2"=w293, "X"=w292, "b"=w291) -> (w294:cluster{"X^2":dbl, "X":dbl, "b":dbl})
            n148 = call "总磷总氮公式写入.vi"("公式"=w294, "error in (no error)"=errorcluster {"status"=FALSE, "code"=0, "source"=""} ("error out"), "量程"=w296, "测量模式"=w298, "测量参数"=w299) -> ("error out"=w289:errorcluster)  [unwired: 6 in]
            n149 = case shown="错误" w289 {
              tunnel: ["写入成功" "写入失败"] -> w290
              frame No Error {
              }
              frame Error {
              }
            }
            n150 = One Button Dialog(message=w290) -> ()  [unwired: 1 in, 1 out]
          }
          frame #1 {
            n151 = Set Occurrence(w303) -> ()
          }
        }
      }
      event "测量精度": Mouse Down {
        n152 = event-data() -> ("CtlRef"=w305:refnum<vi>)  [unwired: 1 in, 7 out]
        n153 = global read "VAR总磷总氮全局变量.vi" "权限等级"() -> (w304:enum16{"一级权限", "二级权限", "三级权限", "超级权限"})
        n154 = case shown="\"二级权限\"..\"超级权限\"" w304 {
          tunnel: w305 -> [_ w309]
          frame "一级权限", Default {
          }
          frame "二级权限".."超级权限" {
            n155 = property class="DigNum (严格)"(reference=w309) -> (reference out=w307:refnum<vi>, "Value"=w308:u16)  [unwired: 1 in, 1 out]
            n156 = call "数字键盘.vi"("OldNumber"=w308) -> ("NewNumber"=w306:dbl)
            n157 = property class="DigNum (严格)"(reference=w307, "Val(Sgnl)"=w306) -> ()  [unwired: 1 in, 2 out]
          }
        }
      }
      event "二次多项式系数", "曲线斜率", "曲线截距": Mouse Down {
        n158 = event-data() -> ("CtlRef"=w311:refnum<vi>)  [unwired: 1 in, 7 out]
        n159 = global read "VAR总磷总氮全局变量.vi" "权限等级"() -> (w310:enum16{"一级权限", "二级权限", "三级权限", "超级权限"})
        n160 = case shown="\"三级权限\", \"超级权限\"" w310 {
          tunnel: w311 -> [_ w315]
          frame "一级权限", Default {
          }
          frame "三级权限", "超级权限" {
            n161 = property class="DigNum (严格)"(reference=w315) -> (reference out=w313:refnum<vi>, "Value"=w314:dbl)  [unwired: 1 in, 1 out]
            n162 = call "数字键盘.vi"("OldNumber"=w314) -> ("NewNumber"=w312:dbl)
            n163 = property class="DigNum (严格)"(reference=w313, "Val(Sgnl)"=w312) -> ()  [unwired: 1 in, 2 out]
          }
        }
      }
      event "盐度补偿值": Mouse Down {
        n164 = event-data() -> ("CtlRef"=w317:refnum<vi>)  [unwired: 1 in, 3 out]
        n165 = global read "VAR总磷总氮全局变量.vi" "权限等级"() -> (w316:enum16{"一级权限", "二级权限", "三级权限", "超级权限"})
        n166 = case shown="\"二级权限\"..\"超级权限\"" w316 {
          tunnel: w317 -> [_ w319]
          frame "一级权限", Default {
          }
          frame "二级权限".."超级权限" {
            n167 = case shown="假" "盐度自动补偿：" {
              tunnel: w319 -> [w323 _]
              frame False {
                n168 = property class="DigNum (严格)"(reference=w323) -> (reference out=w321:refnum<vi>, "Value"=w322:dbl)  [unwired: 1 in, 1 out]
                n169 = call "数字键盘.vi"("OldNumber"=w322) -> ("NewNumber"=w320:dbl)
                n170 = property class="DigNum (严格)"(reference=w321, "Val(Sgnl)"=w320) -> ()  [unwired: 1 in, 2 out]
              }
              frame True {
              }
            }
          }
        }
      }
      event "盐度补偿值": Value Change {
        n171 = event-data() -> ("NewVal"=w324:dbl)  [unwired: 1 in, 5 out]
        n172 = global read "VAR总磷总氮全局变量.vi" "MB session in"() -> (w325:refnum<class "MB_Master.lvclass">)
        n173 = call "盐度补偿值写入.vi"("盐度补偿值"=w324, "MB session in"=w325) -> ()  [unwired: 8 in, 2 out]
      }
      event "跨度值", "零点核查标液浓度", "跨度核查标液浓度", "标样核查标液浓度", "消解时长", "水样测试量程模式", "零点核查量程模式", "跨度核查量程模式", "加标回收量程模式", "标样核查量程模式", "流程路径", "盐度自动补偿：", "IP", "PORT", "请选择串口:", "通信方式选择": Value Change {
        n174 = event-data() -> ()  [unwired: 1 in, 6 out]
        n175 = global read "VAR总磷总氮全局变量.vi" "权限等级"() -> (w327:enum16{"一级权限", "二级权限", "三级权限", "超级权限"})
        n176 = case shown="\"二级权限\"..\"超级权限\"" w327 {
          tunnel: w328 -> [_ w330]
          tunnel: w326 -> [w329 _]
          frame "一级权限", Default {
            n177 = Set Occurrence(w329) -> ()
          }
          frame "二级权限".."超级权限" {
            n178 = flat-sequence {
              tunnel: w330 -> [w350]
              frame #0 {
                n179 = property class="Ring (严格)"(reference=w350) -> ("Value"=w349:u16)  [unwired: 1 in, 2 out]
                n180 = global write "总磷总氮断电保存全局变量.vi" "PORT"("PORT") -> ()
                n181 = global write "总磷总氮断电保存全局变量.vi" "IP"("IP") -> ()
                n182 = global write "总磷总氮断电保存全局变量.vi" "流程路径"("流程路径") -> ()
                n183 = local read "盐度自动补偿："() -> (w336:bool)
                n184 = local read "通信方式选择"() -> (w332:enum16{"串口", "TCP"})
                n185 = global write "总磷总氮断电保存全局变量.vi" "VISA Resource"("请选择串口:") -> ()
                n186 = global write "总磷总氮断电保存全局变量.vi" "MB通信方式选择"(w332) -> ()
                n187 = global write "总磷总氮断电保存全局变量.vi" "盐度自动补偿："(w336) -> ()
                n188 = Bundle("水样测试量程模式"="水样测试量程模式", "零点核查量程模式"="零点核查量程模式", "跨度核查量程模式"="跨度核查量程模式", "加标回收量程模式"="加标回收量程模式", "标样核查量程模式"="标样核查量程模式") -> (w338:T9)  [unwired: 1 in]
                n189 = global read "总磷总氮断电保存全局变量.vi" "质控参数设置"() -> (w344:T10)
                n190 = local read "消解时长"() -> (w331:dbl)
                n191 = To Unsigned Word Integer(number=w338) -> (unsigned 16bit integer=w337:T11)
                n192 = case shown="1" w349 {
                  tunnel: "跨度值" -> [_ w357 w365 w372 w379 w386 w393 w400 w407 w414]
                  tunnel: "标样核查标液浓度" -> [_ w354 w362 w369 w376 w383 w390 w397 w404 w411]
                  tunnel: "跨度核查标液浓度" -> [_ w355 w363 w370 w377 w384 w391 w398 w405 w412]
                  tunnel: "零点核查标液浓度" -> [_ w356 w364 w371 w378 w385 w392 w399 w406 w413]
                  tunnel: w344 -> [_ w359 w367 w374 w381 w388 w395 w402 w409 w416]
                  tunnel: w337 -> [_ w353 w361 w368 w375 w382 w389 w396 w403 _]
                  tunnel: w331 -> [_ w352 w360 _ _ _ _ _ _ w410]
                  frame 0, Default {
                  }
                  frame 1 {
                    n193 = global write "总磷总氮断电保存全局变量.vi" "总氮消解时长"(w352) -> ()
                    n194 = global write "总磷总氮断电保存全局变量.vi" "总磷自动测试量程配置"(w353) -> ()
                    n195 = Bundle By Name(cluster=w359, "总磷跨度值"=w357, "总磷零点标准液浓度"=w356, "总磷跨度标准液浓度"=w355, "总磷标准液标准浓度"=w354) -> (w358:T10)
                    n196 = global write "总磷总氮断电保存全局变量.vi" "质控参数设置"(w358) -> ()
                  }
                  frame 2 {
                    n197 = global write "总磷总氮断电保存全局变量.vi" "总氮消解时长"(w360) -> ()
                    n198 = global write "总磷总氮断电保存全局变量.vi" "总氮自动测试量程配置"(w361) -> ()
                    n199 = Bundle By Name(cluster=w367, "总氮跨度值"=w365, "总氮零点标准液浓度"=w364, "总氮跨度标准液浓度"=w363, "总氮标准液标准浓度"=w362) -> (w366:T10)
                    n200 = global write "总磷总氮断电保存全局变量.vi" "质控参数设置"(w366) -> ()
                  }
                  frame 3 {
                    n201 = global write "总磷总氮断电保存全局变量.vi" "氨氮自动测试量程配置"(w368) -> ()
                    n202 = Bundle By Name(cluster=w374, "氨氮跨度值"=w372, "氨氮零点标准液浓度"=w371, "氨氮跨度标准液浓度"=w370, "氨氮标准液标准浓度"=w369) -> (w373:T10)
                    n203 = global write "总磷总氮断电保存全局变量.vi" "质控参数设置"(w373) -> ()
                  }
                  frame 4 {
                    n204 = Bundle By Name(cluster=w381, "磷酸盐跨度值"=w379, "磷酸盐零点标准液浓度"=w378, "磷酸盐跨度标准液浓度"=w377, "磷酸盐标准液标准浓度"=w376) -> (w380:T10)
                    n205 = global write "总磷总氮断电保存全局变量.vi" "磷酸盐自动测试量程配置"(w375) -> ()
                    n206 = global write "总磷总氮断电保存全局变量.vi" "质控参数设置"(w380) -> ()
                  }
                  frame 5 {
                    n207 = global write "总磷总氮断电保存全局变量.vi" "硝氮自动测试量程配置"(w382) -> ()
                    n208 = Bundle By Name(cluster=w388, "硝氮跨度值"=w386, "硝氮零点标准液浓度"=w385, "硝氮跨度标准液浓度"=w384, "硝氮标准液标准浓度"=w383) -> (w387:T10)
                    n209 = global write "总磷总氮断电保存全局变量.vi" "质控参数设置"(w387) -> ()
                  }
                  frame 6 {
                    n210 = Bundle By Name(cluster=w395, "亚硝氮跨度值"=w393, "亚硝氮零点标准液浓度"=w392, "亚硝氮跨度标准液浓度"=w391, "亚硝氮标准液标准浓度"=w390) -> (w394:T10)
                    n211 = global write "总磷总氮断电保存全局变量.vi" "亚硝氮自动测试量程配置"(w389) -> ()
                    n212 = global write "总磷总氮断电保存全局变量.vi" "质控参数设置"(w394) -> ()
                  }
                  frame 7 {
                    n213 = Bundle By Name(cluster=w402, "硅酸盐跨度值"=w400, "硅酸盐零点标准液浓度"=w399, "硅酸盐跨度标准液浓度"=w398, "硅酸盐标准液标准浓度"=w397) -> (w401:T10)
                    n214 = global write "总磷总氮断电保存全局变量.vi" "硅酸盐自动测试量程配置"(w396) -> ()
                    n215 = global write "总磷总氮断电保存全局变量.vi" "质控参数设置"(w401) -> ()
                  }
                  frame 8 {
                    n216 = Bundle By Name(cluster=w409, "硫化物跨度值"=w407, "硫化物零点标准液浓度"=w406, "硫化物跨度标准液浓度"=w405, "硫化物标准液标准浓度"=w404) -> (w408:T10)
                    n217 = global write "总磷总氮断电保存全局变量.vi" "硫化物自动测试量程配置"(w403) -> ()
                    n218 = global write "总磷总氮断电保存全局变量.vi" "质控参数设置"(w408) -> ()
                  }
                  frame 22 {
                    n219 = global write "总磷总氮断电保存全局变量.vi" "CODcr消解时长"(w410) -> ()
                    n220 = Bundle By Name(cluster=w416, "COD跨度值"=w414, "COD零点标准液浓度"=w413, "COD跨度标准液浓度"=w412, "COD标准液标准浓度"=w411) -> (w415:T10)
                    n221 = global write "总磷总氮断电保存全局变量.vi" "质控参数设置"(w415) -> ()
                  }
                }
              }
              frame #1 {
                n222 = call "配置写入.vi"() -> ()  [unwired: 11 in, 1 out]
              }
            }
          }
        }
      }
      event "通讯连接": Value Change {
        n223 = event-data() -> ("NewVal"=w417:bool)  [unwired: 1 in, 5 out]
        n224 = Flush Queue(queue=w418) -> (queue out=w419:refnum<queue>)  [unwired: 1 in, 2 out]
        n225 = case shown="真" w417 {
          tunnel: w419 -> [w420 w422]
          frame False {
            n226 = Enqueue Element(queue=w420, element=cluster{"命令":string, "data":variant} {"命令"="停用模块", "data"=variant} ("元素")) -> ()  [unwired: 2 in, 3 out]
          }
          frame True {
            n227 = Enqueue Element(queue=w422, element=cluster{"命令":string, "data":variant} {"命令"="启用模块", "data"=variant} ("元素")) -> ()  [unwired: 2 in, 3 out]
          }
        }
      }
    }
  }
  n228 = while {
    tunnel: w8 -> [w434]
    tunnel: w2 -> [w433]
    tunnel: w3 -> [w432]
    tunnel: w1 -> [w431]
    stop <- FALSE stop-if-true
    n229 = Wait on Occurrence(2:w431) -> (0:w424:bool)  [unwired: 2 in]
    n230 = flat-sequence {
      tunnel: w434 -> [w441]
      tunnel: w433 -> [w440]
      tunnel: w432 -> [w439]
      tunnel: [w438] -> w427
      tunnel: [w437] -> w426
      tunnel: [w436] -> w425
      tunnel: w424 -> [_]
      frame #0 {
        n231 = property class="Enum (严格)"(reference=w439) -> ("Value"=w436:enum16{"水样测量", "零点核查", "跨度核查", "标样核查", "加标回收"})  [unwired: 1 in, 2 out]
        n232 = property class="Enum (严格)"(reference=w440) -> ("Value"=w437:enum16{"低量程", "高量程"})  [unwired: 1 in, 2 out]
        n233 = property class="Ring (严格)"(reference=w441) -> ("Value"=w438:u16)  [unwired: 1 in, 2 out]
      }
    }
    n234 = flat-sequence {
      tunnel: [w455] -> w430
      tunnel: [w463] -> w429
      tunnel: [w454] -> w428
      tunnel: w427 -> [w455]
      tunnel: w426 -> [w463]
      tunnel: w425 -> [w454]
      tunnel: w430 -> [w528]
      tunnel: w429 -> [w529]
      tunnel: w428 -> [w530]
      frame #0 {
        n235 = global read "总磷总氮断电保存全局变量.vi" "PORT"() -> (w450:string)
        n236 = global read "总磷总氮断电保存全局变量.vi" "IP"() -> (w451:string)
        n237 = local write "IP"(w451) -> ()
        n238 = local write "PORT"(w450) -> ()
        n239 = global read "总磷总氮断电保存全局变量.vi" "流程路径"() -> (w452:path)
        n240 = local write "流程路径"(w452) -> ()
        n241 = global read "总磷总氮断电保存全局变量.vi" "MB通信方式选择"() -> (w449:enum16{"串口", "TCP"})
        n242 = global read "总磷总氮断电保存全局变量.vi" "VISA Resource"() -> (w448:refnum<visa-resource-name>)
        n243 = global read "总磷总氮断电保存全局变量.vi" "盐度自动补偿："() -> (w453:bool)
        n244 = global read "总磷总氮断电保存全局变量.vi" "质控参数设置"() -> (w446:T10)
        n245 = local write "通信方式选择"(w449) -> ()
        n246 = case shown="1" w455 {
          tunnel: [_ w470 w477 w483 w489 w495 w501 w507 w513 w520] -> w456
          tunnel: [_ w469 w476 _ _ _ _ _ _ w519] -> w447
          tunnel: w446 -> [_ w468 w475 w482 w488 w494 w500 w506 w512 w518]
          tunnel: [_ w467 w474 w481 w487 w493 w499 w505 w511 w517] -> w445
          tunnel: [_ w466 w473 w480 w486 w492 w498 w504 w510 w516] -> w444
          tunnel: [_ w465 w472 w479 w485 w491 w497 w503 w509 w515] -> w443
          tunnel: [_ w464 w471 w478 w484 w490 w496 w502 w508 w514] -> w442
          frame Default {
          }
          frame 1 {
            n247 = Unbundle By Name(w468) -> ("总磷跨度值"=w467:dbl, "总磷零点标准液浓度"=w466:dbl, "总磷跨度标准液浓度"=w465:dbl, "总磷标准液标准浓度"=w464:dbl)
            n248 = global read "总磷总氮断电保存全局变量.vi" "总磷自动测试量程配置"() -> (w470:T12)
            n249 = global read "总磷总氮断电保存全局变量.vi" "总磷消解时长"() -> (w469:dbl)
          }
          frame 2 {
            n250 = Unbundle By Name(w475) -> ("总氮跨度值"=w474:dbl, "总氮零点标准液浓度"=w473:dbl, "总氮跨度标准液浓度"=w472:dbl, "总氮标准液标准浓度"=w471:dbl)
            n251 = global read "总磷总氮断电保存全局变量.vi" "总氮自动测试量程配置"() -> (w477:T12)
            n252 = global read "总磷总氮断电保存全局变量.vi" "总氮消解时长"() -> (w476:dbl)
          }
          frame 3 {
            n253 = Unbundle By Name(w482) -> ("氨氮跨度值"=w481:dbl, "氨氮零点标准液浓度"=w480:dbl, "氨氮跨度标准液浓度"=w479:dbl, "氨氮标准液标准浓度"=w478:dbl)
            n254 = global read "总磷总氮断电保存全局变量.vi" "氨氮自动测试量程配置"() -> (w483:T12)
          }
          frame 4 {
            n255 = Unbundle By Name(w488) -> ("磷酸盐跨度值"=w487:dbl, "磷酸盐零点标准液浓度"=w486:dbl, "磷酸盐跨度标准液浓度"=w485:dbl, "磷酸盐标准液标准浓度"=w484:dbl)
            n256 = global read "总磷总氮断电保存全局变量.vi" "磷酸盐自动测试量程配置"() -> (w489:T12)
          }
          frame 5 {
            n257 = Unbundle By Name(w494) -> ("硝氮跨度值"=w493:dbl, "硝氮零点标准液浓度"=w492:dbl, "硝氮跨度标准液浓度"=w491:dbl, "硝氮标准液标准浓度"=w490:dbl)
            n258 = global read "总磷总氮断电保存全局变量.vi" "硝氮自动测试量程配置"() -> (w495:T12)
          }
          frame 6 {
            n259 = Unbundle By Name(w500) -> ("亚硝氮跨度值"=w499:dbl, "亚硝氮零点标准液浓度"=w498:dbl, "亚硝氮跨度标准液浓度"=w497:dbl, "亚硝氮标准液标准浓度"=w496:dbl)
            n260 = global read "总磷总氮断电保存全局变量.vi" "亚硝氮自动测试量程配置"() -> (w501:T12)
          }
          frame 7 {
            n261 = Unbundle By Name(w506) -> ("硅酸盐跨度值"=w505:dbl, "硅酸盐零点标准液浓度"=w504:dbl, "硅酸盐跨度标准液浓度"=w503:dbl, "硅酸盐标准液标准浓度"=w502:dbl)
            n262 = global read "总磷总氮断电保存全局变量.vi" "硅酸盐自动测试量程配置"() -> (w507:T12)
          }
          frame 8 {
            n263 = Unbundle By Name(w512) -> ("硫化物跨度值"=w511:dbl, "硫化物零点标准液浓度"=w510:dbl, "硫化物跨度标准液浓度"=w509:dbl, "硫化物标准液标准浓度"=w508:dbl)
            n264 = global read "总磷总氮断电保存全局变量.vi" "硫化物自动测试量程配置"() -> (w513:T12)
          }
          frame 22 {
            n265 = Unbundle By Name(w518) -> ("COD跨度值"=w517:dbl, "COD零点标准液浓度"=w516:dbl, "COD跨度标准液浓度"=w515:dbl, "COD标准液标准浓度"=w514:dbl)
            n266 = global read "总磷总氮断电保存全局变量.vi" "COD自动测试量程配置"() -> (w520:T12)
            n267 = global read "总磷总氮断电保存全局变量.vi" "CODcr消解时长"() -> (w519:dbl)
          }
        }
        "消解时长" <- w447
        n268 = local write "请选择串口:"(w448) -> ()
        n269 = local write "盐度自动补偿："(w453) -> ()
        n270 = local write "跨度值"(w445) -> ()
        n271 = local write "零点核查标液浓度"(w444) -> ()
        n272 = local write "标样核查标液浓度"(w442) -> ()
        n273 = To Unsigned Word Integer(number=w456) -> (unsigned 16bit integer=w457:T13)
        n274 = local write "跨度核查标液浓度"(w443) -> ()
        n275 = Unbundle By Name(w457) -> ("水样测试量程模式"=w458:u16, "空白核查量程模式"=w460:u16, "跨度核查量程模式"=w461:u16, "加标回收量程模式"=w462:u16, "标样核查量程模式"=w459:u16)
        n276 = local write "标样核查量程模式"(w459) -> ()
        n277 = local write "水样测试量程模式"(w458) -> ()
        n278 = local write "零点核查量程模式"(w460) -> ()
        n279 = local write "跨度核查量程模式"(w461) -> ()
        n280 = local write "加标回收量程模式"(w462) -> ()
      }
      frame #1 {
        n281 = call "总磷总氮量程读取.vi"("测量参数"=w528) -> ("error out"=w535:errorcluster, "量程参数读取"=w543:T5)  [unwired: 9 in]
        n282 = Unbundle By Name(w543) -> ("测量精度"=→"测量精度":u16, "检出限"=→"检出限":dbl, "上限"=→"量程上限":dbl, "下限"=→"量程下限":dbl, "阈值（低->高）"=→"阈值（低->高）":dbl, "阈值（高->低）"=→"阈值（高->低）":dbl, "稀释度"=→"稀释度":dbl)
        n283 = global read "VAR总磷总氮全局变量.vi" "MB session in"() -> (w524:refnum<class "MB_Master.lvclass">)
        n284 = call "总磷总氮公式读取.vi"("error in (no error)"=w535, "量程"=w529, "测量模式"=w530, "测量参数"=w528) -> ("error out"=w521:errorcluster, "公式"=w534:cluster{"X^2":dbl, "X":dbl, "b":dbl})  [unwired: 6 in]
        n285 = Unbundle By Name(w534) -> ("X^2"=→"二次多项式系数":dbl, "X"=→"曲线斜率":dbl, "b"=→"曲线截距":dbl)
        n286 = call "读取外设配置.vi"("error in (no error)"=w521, "MB session in"=w524) -> ("error out"=w523:errorcluster, "外设配置"=w526:T6, "MB session out"=w527:refnum<class "MB_Master.lvclass">)  [unwired: 7 in]
        n287 = Unbundle By Name(w526) -> ("消解温度下限"=→"消解温度":sgl)
        n288 = call "盐度补偿值读取.vi"("Error in"=w523, "MB session in"=w527) -> ("盐度补偿值"=→"盐度补偿值":sgl)  [unwired: 7 in, 2 out]
      }
      frame #2 {
        n289 = Format Date/Time String() -> (date/time string=→"数据刷新时间":string)  [unwired: 3 in]
      }
    }
  }
